vi "PID.vi"(1 "Present Value":dbl=15.0 format="%.2f", 2 "Previous Scan Value":dbl format="%.2f", 3 "Setpoint":dbl=15.0 format="%.2f") -> (0 "Dem Output":dbl format="%.2f")   [LabVIEW 2016]
uses:
  <vilib>/Analysis/NI_AALPro.lvlib
panel:
  out "Derivative":dbl(graph)
  out "Integral":dbl(graph)
  out "Proportional":dbl(graph)
  out "Error":dbl(graph)
  in  "Error DeadBand":dbl
  in  "O/P deadband":dbl=0.2 format="%.2f"
  in  "Kp Deadband":dbl format="%.2f"
  in  "Derivative History":i32=35
  out "deadbanded error":dbl format="%.2f"
  in  "P":bool=TRUE
  in  "D":bool=TRUE
  in  "I":bool=TRUE
  in  "Manual Demand":dbl min=0.0 max=100.0 format="%.2f"
  in  "Manual Override":bool
  out "Control Sum":dbl format="%.2f"
  out "error differential":dbl format="%.5f"
  out "error integral":dbl format="%.2f"
  in  "Kd":dbl=2000.0 format="%.2f"
  in  "Ki":dbl=0.035 format="%.3f"
  in  "Kp":dbl=5.0 format="%.2f"
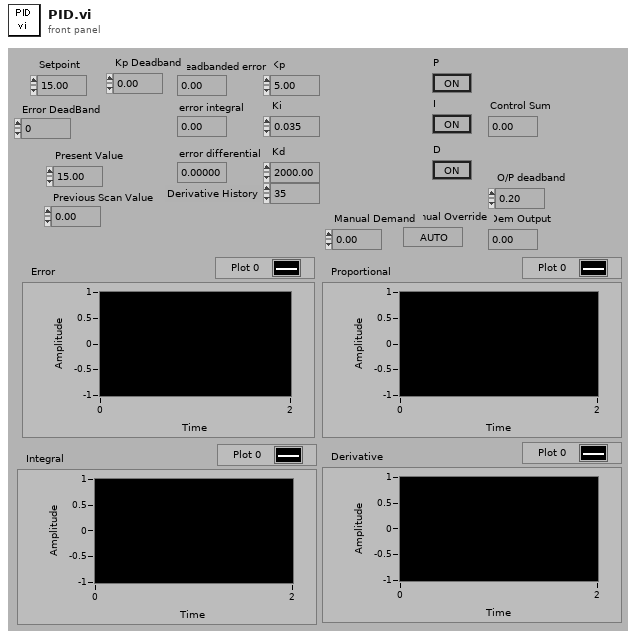
[diagram p1: front panel]
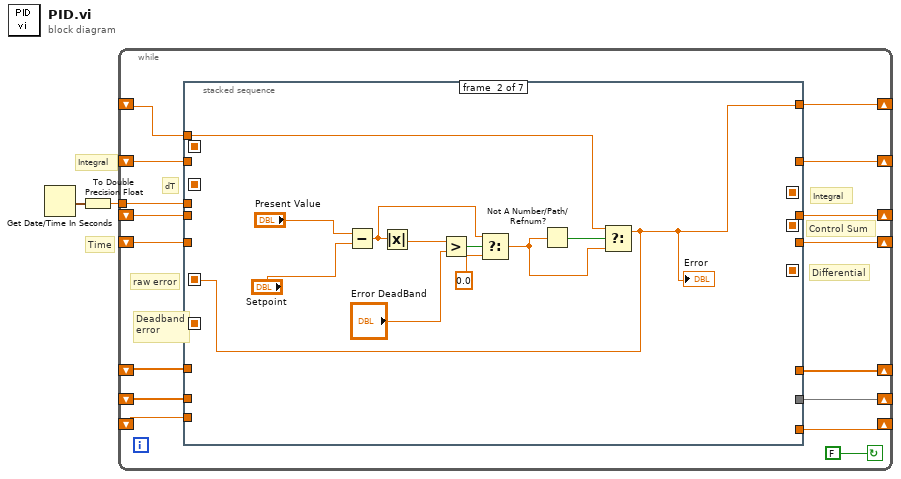
[diagram p0: block diagram]
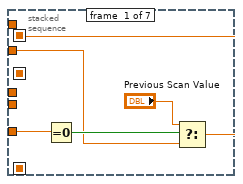
[diagram p2: hidden frame]
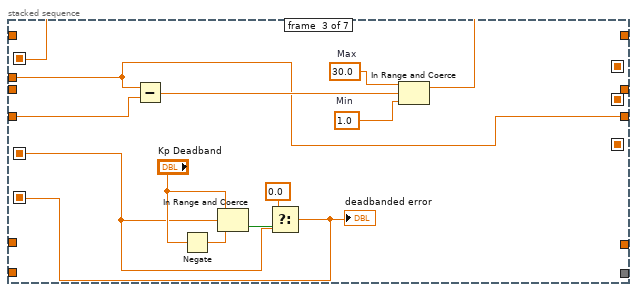
[diagram p3: hidden frame]
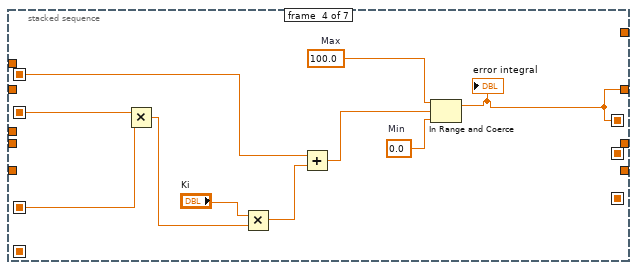
[diagram p4: hidden frame]
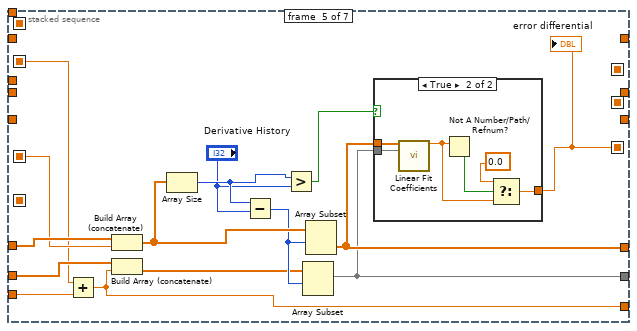
[diagram p5: hidden frame]
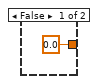
[diagram p6: hidden frame]
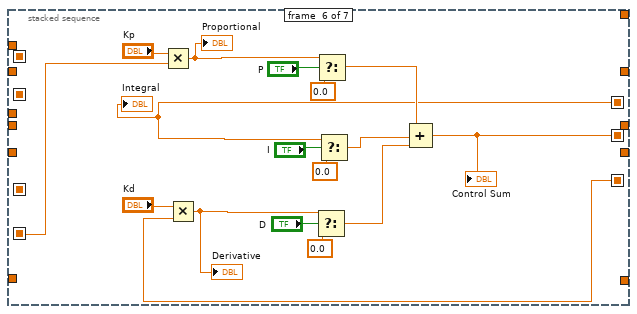
[diagram p7: hidden frame]
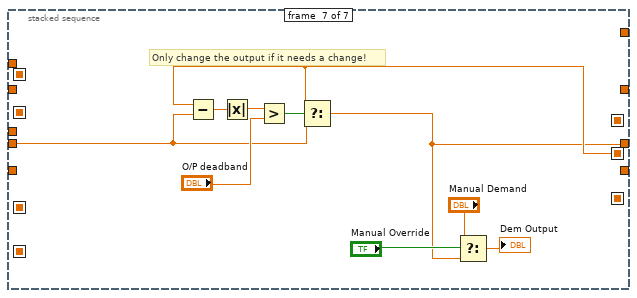
[diagram p8: hidden frame]
diagram:
  # "Integral"
  # "Time"
  n1 = Get Date/Time In Seconds() -> (seconds since 1Jan1904=w1:timestamp)
  n2 = To Double Precision Float(number=w1) -> (double precision float=w2:dbl)
  n3 = while {
    shift-left: _ -> [w5]
    shift-right: [w4] -> _
    shift-left: _ -> [w7]
    shift-right: [w6] -> _
    shift-left: _ -> [w9]
    shift-right: [w8] -> _
    tunnel: w2 -> [w14]
    shift-left: _ -> [w11]
    shift-right: [w10] -> _
    shift-left: _ -> [w13]
    shift-right: [w12] -> _
    shift-left: _ -> [w15]
    shift-right: [w16] -> _
    shift-left: _ -> [w18]
    shift-right: [w17] -> _
    stop <- FALSE continue-if-true
    # "Control Sum"
    # "raw error"
    # "Differential"
    # "Integral"
    # "Deadband\nerror"
    # "dT"
    n4 = stacked-sequence {
      seq-local: [_ _ w35 _ _ _ _] -> [_ _ _ w56 w62 _ _]
      seq-local: [_ _ w44 _ _ _ _] -> [_ _ _ _ _ w83 _]
      seq-local: [_ _ _ _ w64 _ _] -> [_ _ _ _ _ w82 _]
      seq-local: [_ _ _ w51 _ _ _] -> [_ _ _ _ _ w80 _]
      seq-local: [_ w24 _ _ _ _ _] -> [_ _ w36 w53 w65 _ _]
      seq-local: [_ _ _ _ _ w86 _] -> [_ _ _ _ _ _ w99]
      seq-local: [w19 _ _ _ _ _ _] -> [_ _ _ w47 _ _ _]
      tunnel: w18 -> [w23 _ w41 _ _ _ _]
      tunnel: [_ _ w39 _ _ _ _] -> w17
      tunnel: [_ _ _ w51 _ _ _] -> w16
      tunnel: w15 -> [w20 _ _ _ _ _ _]
      tunnel: w14 -> [_ _ w39 _ _ _ _]
      tunnel: w13 -> [_ _ _ _ w71 _ _]
      tunnel: [_ _ _ _ w66 _ _] -> w12
      tunnel: w11 -> [_ _ _ _ w70 _ _]
      tunnel: [_ _ _ _ w63 _ _] -> w10
      tunnel: w9 -> [_ _ _ _ _ _ w97]
      tunnel: [_ _ _ _ _ _ w96] -> w8
      tunnel: w7 -> [_ _ _ _ w61 _ _]
      tunnel: [_ _ _ _ w60 _ _] -> w6
      tunnel: w5 -> [_ w31 _ _ _ _ _]
      tunnel: [_ w24 _ _ _ _ _] -> w4
      frame #0 {
        n5 = Equal To 0?(x=w23) -> (x = 0?=w22:bool)
        n6 = Select(t="Previous Scan Value", s=w22, f=w20) -> (s? t:f=w19:dbl)
      }
      frame #1 {
        n7 = Subtract(x="Present Value", y="Setpoint") -> (x-y=w26:dbl)
        n8 = Absolute Value(x=w26) -> (abs(x)=w30:dbl)
        n9 = Greater?(x=w30, y="Error DeadBand") -> (0:w28:bool)
        n10 = Select(t=w26, s=w28, f=0.0 ("t")) -> (s? t:f=w27:dbl)
        n11 = Not A Number/Path/Refnum?(number/path/refnum=w27) -> (NaN/Path/Refnum?=w32:bool)
        n12 = Select(t=w31, s=w32, f=w27) -> (s? t:f=w24:dbl)
        "Error" <- w24
      }
      frame #2 {
        w42 = 1.0  # Min
        w43 = 30.0  # Max
        n13 = Subtract(x=w39, y=w41) -> (x-y=w40:dbl)
        n14 = Negate(x="Kp Deadband") -> (-x=w38:dbl)
        n15 = In Range and Coerce(upper limit="Kp Deadband", x=w36, lower limit=w38) -> (In Range?=w45:bool)  [unwired: 1 out]
        n16 = Select(t=0.0, s=w45, f=w36) -> (s? t:f=w44:dbl)
        "deadbanded error" <- w44
        n17 = In Range and Coerce(upper limit=w43, x=w40, lower limit=w42) -> (coerced(x)=w35:dbl)  [unwired: 1 out]
      }
      frame #3 {
        w55 = 0.0  # Min
        w50 = 100.0  # Max
        n18 = Multiply(x=w56, y=w53) -> (x*y=w49:dbl)
        n19 = Multiply(x="Ki", y=w49) -> (x*y=w52:dbl)
        n20 = Add(x=w47, y=w52) -> (x+y=w54:dbl)
        n21 = In Range and Coerce(upper limit=w50, x=w54, lower limit=w55) -> (coerced(x)=w51:dbl)  [unwired: 1 out]
        "error integral" <- w51
      }
      frame #4 {
        n22 = Add(x=w62, y=w61) -> (x+y=w60:dbl)
        n23 = Build Array (concatenate)(w71, w65) -> (w69:dbl[])
        n24 = Build Array (concatenate)(w70, w60) -> (w67:dbl[])
        n25 = Array Size(array=w69) -> (size(s)=w58:i32)
        n26 = Subtract(x=w58, y="Derivative History") -> (x-y=w68:i32)
        n27 = Greater?(x=w58, y="Derivative History") -> (0:w59:bool)
        n28 = Array Subset(array=w67, index=w68) -> (w63:dbl[])  [unwired: 1 in]
        n29 = Array Subset(array=w69, index=w68) -> (w66:dbl[])  [unwired: 1 in]
        n30 = case shown="True" w59 {
          tunnel: w66 -> [_ w78]
          tunnel: [0.0 ("slope") w77] -> w64
          tunnel: w63 -> [_ w76]
          frame False {
          }
          frame True {
            n31 = call <vilib>:"Linear Fit Coefficients.vi"("Y"=w78, "X"=w76) -> ("slope"=w73:dbl)  [unwired: 3 in, 10 out]
            n32 = Not A Number/Path/Refnum?(number/path/refnum=w73) -> (NaN/Path/Refnum?=w75:bool)
            n33 = Select(t=0.0 ("f"), s=w75, f=w73) -> (s? t:f=w77:dbl)
          }
        }
        "error differential" <- w64
      }
      frame #5 {
        n34 = Multiply(x="Kp", y=w83) -> (x*y=w79:dbl)
        "Proportional" <- w79
        n35 = Multiply(x="Kd", y=w82) -> (x*y=w81:dbl)
        "Derivative" <- w81
        n36 = Select(t=w81, s="D", f=0.0) -> (s? t:f=w88:dbl)
        n37 = Select(t=w79, s="P", f=0.0) -> (s? t:f=w94:dbl)
        n38 = Select(t=w80, s="I", f=0.0) -> (s? t:f=w87:dbl)
        n39 = Compound Arithmetic op=ADD(w94, w87, w88) -> (w86:dbl)
        "Control Sum" <- w86
        "Integral" <- w80
      }
      frame #6 {
        # "Only change the output if it needs a change!"
        n40 = Subtract(x=w99, y=w97) -> (x-y=w102:dbl)
        n41 = Absolute Value(x=w102) -> (abs(x)=w101:dbl)
        n42 = Greater?(x=w101, y="O/P deadband") -> (0:w100:bool)
        n43 = Select(t=w99, s=w100, f=w97) -> (s? t:f=w96:dbl)
        n44 = Select(t="Manual Demand", s="Manual Override", f=w96) -> (s? t:f=→"Dem Output":dbl)
      }
    }
  }
